vi "PCU_Information.vi"(0 ".NET Reference in":refnum<k24>, 11 "error in (no error)":errorcluster) -> (4 "Reference out":refnum<k24>, 6 "Band":string, 8 "FWversion":string, 10 "ProductName":string, 14 "SerialNumber":string, 15 "error out":errorcluster)   [LabVIEW 2017]
uses:
  C:/Users/Ssantec_Test/Documents/Instrument_DLL_Sample_Labview_20250826_Ver1.5.0_x64/DLL/InstrumentDLL.dll
  DLL/InstrumentDLL.dll
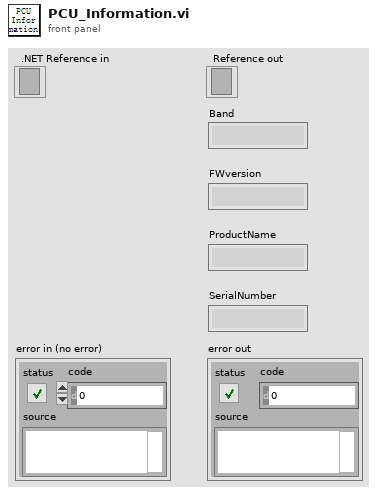
[diagram p1: front panel]
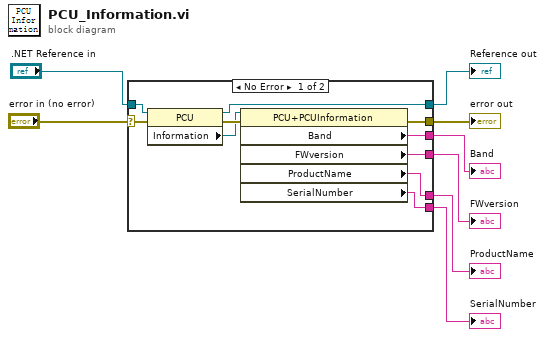
[diagram p0: block diagram]
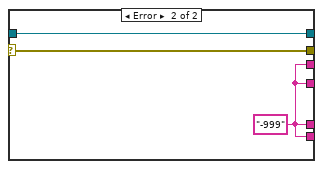
[diagram p2: hidden frame]
diagram:
  n1 = case shown="No Error" "error in (no error)" {
    selector: "error in (no error)" -> [w12 w21]
    tunnel: ".NET Reference in" -> [w17 w19]
    tunnel: [w16 w20] -> w7
    tunnel: [w15 w20] -> w6
    tunnel: [w14 w20] -> w5
    tunnel: [w13 w20] -> w4
    tunnel: [w10 w21] -> w2
    tunnel: [w9 w19] -> w1
    frame No Error {
      n2 = property on="属性节点" class="PCU"(reference=w17, error in=w12) -> (reference out=w9:refnum<k24>, error out=w18:errorcluster, "Information"=w11:refnum<k24>)
      n3 = property on="属性节点" class="PCU+PCUInformation"(reference=w11, error in=w18) -> (error out=w10:errorcluster, "Band"=w16:string, "FWversion"=w14:string, "ProductName"=w15:string, "SerialNumber"=w13:string)  [unwired: 1 out]
    }
    frame Error {
      w20 = "-999" ("Band")
    }
  }
  "Band" <- w7
  "ProductName" <- w6
  "FWversion" <- w5
  "SerialNumber" <- w4
  "error out" <- w2
  "Reference out" <- w1
